vi "Boonton7200_Read_GPIB_Cp.vi"(7 "GPIB Address String":string, 8 "Error In":errorcluster) -> (0 "Error Out":errorcluster, 1 "External bias":dbl, 2 "Conductance":dbl, 3 "Capacitance":dbl, 4 "Raw output":string)   [LabVIEW 2015, in "Boonton7200.lvlib"]
uses:
  Boonton7200.lvlib
  <vilib>/Utility/error.llb/Error Cluster From Error Code.vi
  <vilib>/ErrorRing/Error Ring.xnode
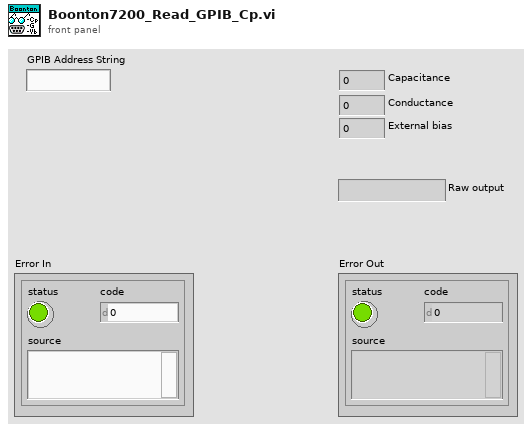
[diagram p1: front panel]
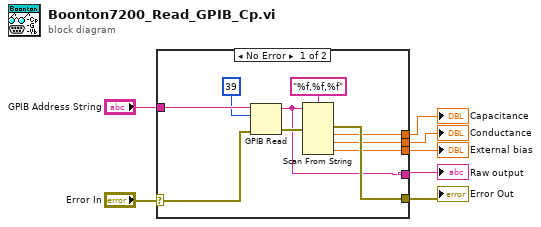
[diagram p0: block diagram]
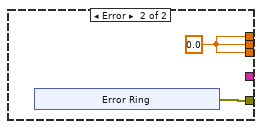
[diagram p2: hidden frame]
diagram:
  n1 = case shown="No Error" "Error In" {
    selector: "Error In" -> [w14 _]
    tunnel: [w12 w18] -> w6
    tunnel: "GPIB Address String" -> [w17 _]
    tunnel: [w11 w19] -> w1
    tunnel: [w10 w19] -> w4
    tunnel: [w9 w19] -> w3
    tunnel: [w8 _] -> w2
    frame No Error {
      n2 = GPIB Read(0:w17, 1:39 ("byte count"), 3:w14) -> (5:w8:string, 7:w15:errorcluster)  [unwired: 2 in, 1 out]
      n3 = Scan From String(format string="%f,%f,%f", input string=w8, error in=w15) -> (error out=w12:errorcluster, output 1=w11:dbl, output 2=w10:dbl, output 3=w9:dbl)  [unwired: 4 in, 2 out]
    }
    frame Error {
      w19 = 0.0
      n4 = xnode "Error Ring"() -> ("error out"=w18:errorcluster)
    }
  }
  "Error Out" <- w6
  "Capacitance" <- w1
  "Conductance" <- w4
  "External bias" <- w3
  "Raw output" <- w2
